vi "Buttons Example.vi"() -> ()   [LabVIEW 2015]
uses:
  ROS/Code/SubVIs/BaxterButtons.ctl
  ROS/Code/SubVIs/DigitalIOComponents.ctl
panel:
  in  "stop":bool
  out "Left ITB":T1
  # "Hitting the long buttons on his wrist toggles the lights on his arms"
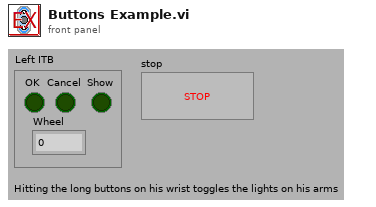
[diagram p1: front panel]
types:
  T1 = cluster{"OK":bool, "Cancel":bool, "Show":bool, "Wheel":u8}
  T2 = typedef "BaxterButtons.ctl" = enum16{"left_itb", "right_itb", "torso_left_itb", "torso_right_itb"}
  T3 = typedef "DigitalIOComponents.ctl" = enum16{"left_lower_cuff", "right_lower_cuff", "left_lower_button", "right_lower_button", "left_upper_button", "right_upper_button", "left_shoulder_button", "right_shoulder_button"}
  T4 = cluster{"Component":T3, "state":i8, "is input only":bool}[]
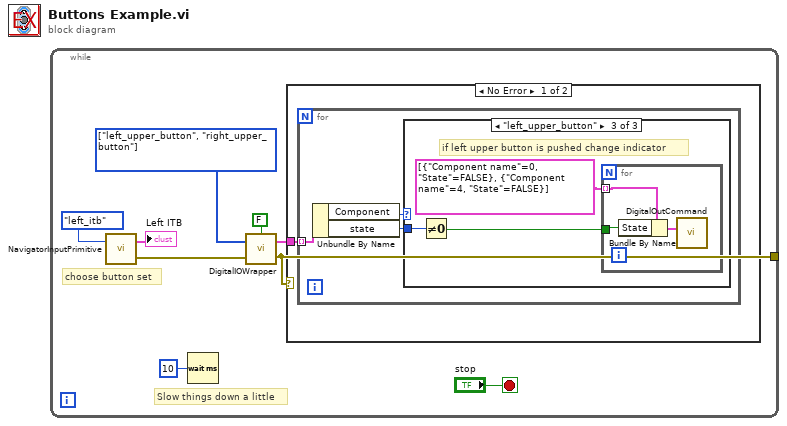
[diagram p0: block diagram]
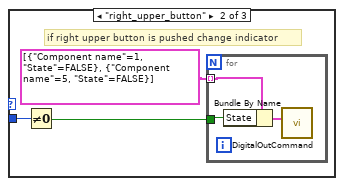
[diagram p3: hidden frame]
diagram:
  n1 = while {
    tunnel: [w2] -> _
    stop <- "stop" stop-if-true
    w4 = T3[] [enum."left_upper_button", enum."right_upper_button"] items=["left_lower_cuff", "right_lower_cuff", "left_lower_button", "right_lower_button", "left_upper_button", "right_upper_button", "left_shoulder_button", "right_shoulder_button"] ("Component IDs")
    # "choose button set"
    # "Slow things down a little"
    n2 = call "NavigatorInputPrimitive.vi"("Component"=BaxterButtons."left_itb") -> ("error out"=w5:errorcluster, "Navigator Inputs"=→"Left ITB":T1)  [unwired: 2 in]
    n3 = Wait (ms)(milliseconds to wait=u32 10) -> ()  [unwired: 1 out]
    n4 = call "DigitalIOWrapper.vi"("error in"=w5, "Component IDs"=w4, "True Only (T)"=FALSE) -> ("error out"=w2:errorcluster, "Changed_IO"=w3:T4)
    n5 = case shown="No Error" w2 {
      tunnel: w3 -> [w10 _]
      frame No Error {
        n6 = for {
          tunnel: w10 -> [w13] mode=indexing
          n7 = Unbundle By Name(w13) -> ("Component"=w12:T3, "state"=w11:i8)
          n8 = case shown="\"left_upper_button\"" w12 {
            tunnel: w11 -> [_ w16 w22]
            frame Default {
            }
            frame "right_upper_button" {
              # "if right upper button is pushed change indicator"
              n9 = Not Equal To 0?(x=w16) -> (x != 0?=w15:bool)
              n10 = for {
                tunnel: w15 -> [w19]
                tunnel: cluster{"Component name":u16, "State":bool}[] [{"Component name"=1, "State"=FALSE}, {"Component name"=5, "State"=FALSE}] -> [w18] mode=indexing
                n11 = Bundle By Name(cluster=w18, "State"=w19) -> (w17:cluster{"Component name":u16, "State":bool})
                n12 = call "DigitalOutCommand.vi"("Parameters"=w17) -> ()  [unwired: 3 in, 1 out]
              }
            }
            frame "left_upper_button" {
              # "if left upper button is pushed change indicator"
              n13 = Not Equal To 0?(x=w22) -> (x != 0?=w21:bool)
              n14 = for {
                tunnel: w21 -> [w25]
                tunnel: cluster{"Component name":u16, "State":bool}[] [{"Component name"=0, "State"=FALSE}, {"Component name"=4, "State"=FALSE}] -> [w24] mode=indexing
                n15 = Bundle By Name(cluster=w24, "State"=w25) -> (w23:cluster{"Component name":u16, "State":bool})
                n16 = call "DigitalOutCommand.vi"("Parameters"=w23) -> ()  [unwired: 3 in, 1 out]
              }
            }
          }
        }
      }
      frame Error {
      }
    }
  }
